vi "Untitled 4.vi"   [LabVIEW 2021]
uses:
  <vilib>/ActorFramework/Self-Addressed Msg/Self-Addressed Msg.lvclass
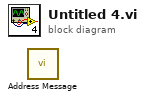
[diagram p0: block diagram]
diagram:
  n1 = call <vilib>:"Address Message.vi"() -> ()  [unwired: 11 in, 1 out]
